vi "VMI_save_IF32_files.vi"(5 "Remote_path\n in":path[](array[path]), 6 "Image Info":T2 {"Centroiding" min=1.0}, 7 "file_path":string, 8 "error in (no error)":errorcluster, 9 "Peak Controls":T1, 10 "FileEnd":string, 11 "file ending":string) -> (0 "error out":errorcluster, 3 "Array":path[](array[path]))   [LabVIEW 2020]
uses:
  Type defs/Image_info.ctl
  Type defs/VMI_peak_out.ctl
  Type defs/Header_infor_IF32.ctl
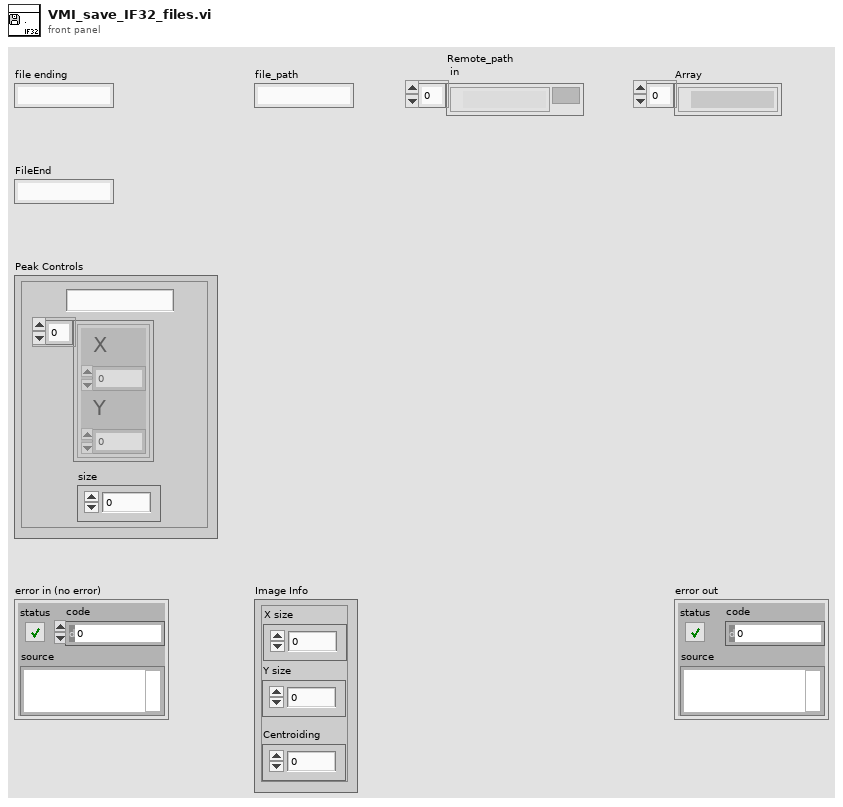
[diagram p1: front panel]
types:
  T1 = typedef "VMI_peak_out.ctl" = cluster{"Peaks":cluster{"X":sgl, "Y":sgl}[], "size":i32, "Title":string}
  T2 = typedef "Image_info.ctl" = cluster{"X size":dbl, "Y size":dbl, "Centroiding":dbl}
  T3 = typedef "Header_infor_IF32.ctl" = cluster{"File Name":string, "Time":string, "Date":string, "Size":string}
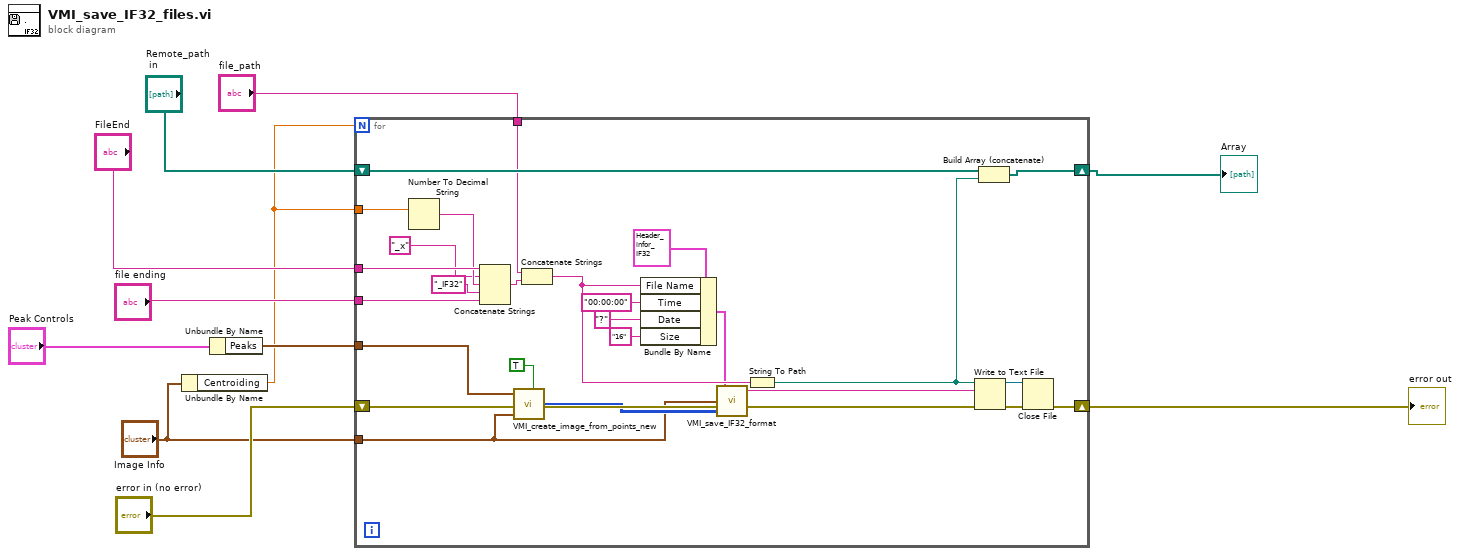
[diagram p0: block diagram]
diagram:
  n1 = Unbundle By Name("Image Info") -> ("Centroiding"=w1:dbl)
  n2 = Unbundle By Name("Peak Controls") -> ("Peaks"=w5:cluster{"X":sgl, "Y":sgl}[])
  n3 = for {
    N: w1 -> [_]
    tunnel: "file_path" -> [w24]
    tunnel: "file ending" -> [w22]
    tunnel: "FileEnd" -> [w14]
    tunnel: w5 -> [w19]
    tunnel: "Image Info" -> [w17]
    shift-right: [w35] -> w10
    shift-left: "error in (no error)" -> [w26]
    shift-right: [w16] -> w2
    shift-left: "Remote_path\n in" -> [w36]
    tunnel: w1 -> [w15]
    n4 = Number To Decimal String(number=w15) -> (decimal integer string=w13:string)  [unwired: 1 in]
    n5 = Concatenate Strings(w14, "_x" ("string"), w13, "_IF32" ("string"), w22) -> (w23:string)
    n6 = call "VMI_create_image_from_points_new.vi"("New Array"=TRUE, "Image Info"=w17, "Points"=w19) -> ("Image Array"=w20:i16[][])  [unwired: 2 in]
    n7 = Concatenate Strings(w24, w23) -> (w32:string)
    n8 = Bundle By Name(cluster=T3 {"File Name"="080916aa", "Time"="Hammer", "Date"="Now", "Size"=""} ("Cluster"), "File Name"=w32, "Time"="00:00:00", "Date"="?", "Size"="16") -> (w31:T3)
    n9 = call "VMI_save_IF32_format.vi"("Image Array"=w20, "Image Info"=w17, "Header Cluster"=w31) -> ("File String"=w25:string)  [unwired: 2 in]
    n10 = String To Path(string=w32) -> (path=w37:path)
    n11 = Write to Text File(file (use dialog)=w37, text=w25, error in=w26) -> (refnum out=w33:refnum<file>, error out=w34:errorcluster)  [unwired: 1 in, 1 out]
    n12 = Build Array (concatenate)(w36, w37) -> (w16:path[])
    n13 = Close File(refnum=w33, error in=w34) -> (error out=w35:errorcluster)  [unwired: 1 out]
  }
  "Array" <- w2
  "error out" <- w10
